vi "Write OVP_Enable.vi"(8 "error in":errorcluster, 10 "OVP_Enable":bool, 11 "PowerSupply in":refnum<class "PowerSupply.lvclass">) -> (0 "error out":errorcluster, 3 "PowerSupply out":refnum<class "PowerSupply.lvclass">)   [LabVIEW 2019, in "PowerSupply.lvlib" / "PowerSupply.lvclass"]
uses:
  Library/PowerSupply.lvclass
  C:/Users/Public/Documents/Development/builds/Instruments/Instruments.lvlibp/Library/Instruments.lvclass
  Library/PowerSupply.lvclass/PowerSupply.ctl
  Read Settings.vi
  Write Settings.vi
  builds/Instruments/Instruments.lvlibp/Accessors/Command with Logging.vi
  builds/Engine/Engine.lvlibp/Project/Engine.lvclass
  builds/Instruments/Instruments.lvlibp/Library/Instruments.lvclass
  builds/Instruments/Instruments.lvlibp/Private/Polymorphic/Special/Event from Boolean.vi
  builds/Instruments/Instruments.lvlibp
  C:/Users/Public/Documents/Development/builds/Tools/Config.lvlibp/Config.lvclass
  C:/Users/Public/Documents/Development/builds/Engine/Engine.lvlibp/Project/Engine.lvclass
  C:/Users/Public/Documents/Development/builds/Engine/Panel Manager.lvlibp/Panel Actor/Panel Actor.lvclass
  C:/Users/Public/Documents/Development/builds/Engine/Monitored Actor.lvlibp/Monitored Actor/Monitored Actor/Monitored Actor.lvclass
  C:/Users/Public/Documents/Development/builds/Engine/Actor Framework.lvlibp/1abvi3w/vi.lib/ActorFramework/Actor/Actor.lvclass
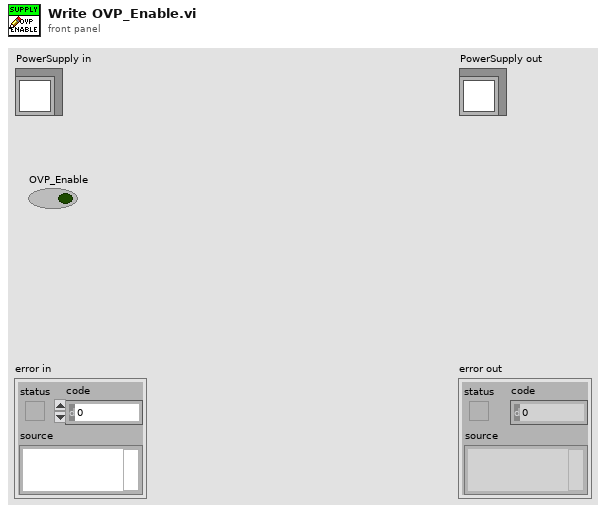
[diagram p1: front panel]
types:
  T1 = typedef "PowerSupply.lvlib/PowerSupply.lvclass/Settings.ctl" = cluster{"Voltage":dbl, "Current":dbl, "Output":bool, "OverVolt_Protect":dbl, "OverCurrent_Protect":dbl, "OVP":bool, "OCP":bool, "Interlock":bool, "Volt_Ramp":dbl, "Current_Ramp":dbl, "Sense Point":T2, "OCP Mode":T3}
  T2 = typedef "PowerSupply.lvlib/PowerSupply.lvclass/Sense Point.ctl" = enum16{"Local", "Remote"}
  T3 = typedef "PowerSupply.lvlib/PowerSupply.lvclass/OCP Mode.ctl" = enum16{"Shutdown", "Foldback"}
  T4 = cluster{"Timestamp":timestamp, "Description":string, "Data":string}
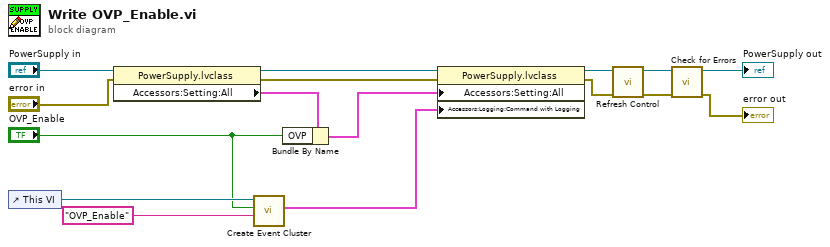
[diagram p0: block diagram]
diagram:
  n1 = control-ref of="This VI"() -> (w4:refnum<vi>)
  n2 = property class="PowerSupply.lvclass"(reference="PowerSupply in", error in="error in") -> (reference out=w16:refnum<class "PowerSupply.lvclass">, error out=w6:errorcluster, "Accessors:Setting:All"=w8:T1)
  n3 = call-poly "Create Event Cluster.vi"("Name"="OVP_Enable", "Value"="OVP_Enable", "VI Refnum"=w4) -> ("Event Data"=w2:T4)  [unwired: 8 in]
  n4 = Bundle By Name(cluster=w8, "OVP"="OVP_Enable") -> (w7:T1)
  n5 = property class="PowerSupply.lvclass"(reference=w16, error in=w6, "Accessors:Setting:All"=w7, "Accessors:Logging:Command with Logging"=w2) -> (reference out=w15:refnum<class "PowerSupply.lvclass">, error out=w5:errorcluster)
  n6 = call "Refresh Control.vi"("error in"=w5, "PowerSupply in"=w15) -> ("error out"=w14:errorcluster, "PowerSupply out"=w13:refnum<class "PowerSupply.lvclass">)  [unwired: 8 in]
  n7 = call "Check for Errors.vi"("error in"=w14, "Engine in"=w13) -> ("error out"=→"error out":errorcluster, "Engine out"=→"PowerSupply out":refnum<class "PowerSupply.lvclass">)  [unwired: 8 in]
